vi "ProyectoBioCuinique Alpha 4.0.vi"() -> ()   [LabVIEW 2021]
uses:
  <vilib>/Utility/NIReport.llb/Report Type.ctl
  <extravilib>/ChannelInstances/Tag-dbl/Read With Abort.vi
  <extravilib>/ChannelInstances/Tag-bool/Read With Abort.vi
  <extravilib>/ChannelInstances/Tag-bool/Write With Abort.vi
  <extravilib>/ChannelInstances/Tag-dbl/Write With Abort.vi
  <vilib>/Instr/_visa.llb/VISA Configure Serial Port (Instr).vi
  <vilib>/MakerHub/LINX/Public/Utilities/Open Serial.vi
  <extravilib>/ChannelInstances/Tag-dbl/Instantiate.vi
  <extravilib>/ChannelInstances/Tag-bool/Instantiate.vi
  <extravilib>/ChannelInstances/Tag-dbl/EndpointRead.vi
  <vilib>/addons/_office/excel.llb/Excel Easy Table (str).vi
  <extravilib>/ChannelInstances/Tag-bool/EndpointRead.vi
  <extravilib>/ChannelInstances/Tag-bool/Endpoint.vi
  <extravilib>/ChannelInstances/Tag-dbl/Endpoint.vi
  <vilib>/Utility/NIReport.llb/NI_report.lvclass
  <vilib>/LabVIEW Interface for Arduino/LabVIEW Interface for Arduino.lvlib
  <vilib>/MakerHub/LINX/LMH-LINX.lvlib
  <vilib>/Utility/NIReport.llb/NI_ReportGenerationCore.lvlib
  <vilib>/addons/_office/NI_ReportGenerationToolkit.lvlib
  <vilib>/Utility/NIReport.llb/Excel/NI_Excel.lvclass
  <vilib>/MakerHub/LINX/Public/Sensors/Distance/Ultrasonic/Ultrasonic.lvlib
  <extravilib>/ChannelInstances/Tag-bool.lvlib
  <extravilib>/ChannelInstances/Tag-dbl.lvlib
panel:
  out "HUMEDAD SUELO":dbl(knob) scale=0.0..255.0
  out "TEMPERATURA":dbl(slide) scale=0.0..100.0
  out "HUMEDAD SUELO":dbl
  in  "Serial Port":refnum<visa-resource-name>="N/A"
  in  "template (empty)":path
  in  "Pin Bomba 1":u8
  in  "Pin Valvula 1":u8
  in  "Pin Valvula 2":u8
  out "HUMEDAD RELATIVA":dbl
  in  "VISA resource name":refnum<visa-resource-name>
  out "TEMPERATURA":dbl
  out "HUMEDAD RELATIVA":dbl(knob) scale=0.0..255.0
  out "Centimeters":dbl
  out "Slide":dbl(slide) scale=0.0..500.0
  out "BOMBA (11)":bool
  in  "Boolean 4":bool
  out "VALVULA (6)":bool
  in  "Boolean":bool
  out "VALVULA (5)":bool
  in  "stop":bool
  in  "VISA resource":refnum<visa-resource-name>
  # "VÁLVULA 1"
  # "BOMBA DE AGUA"
  # "VÁLVULA 2"
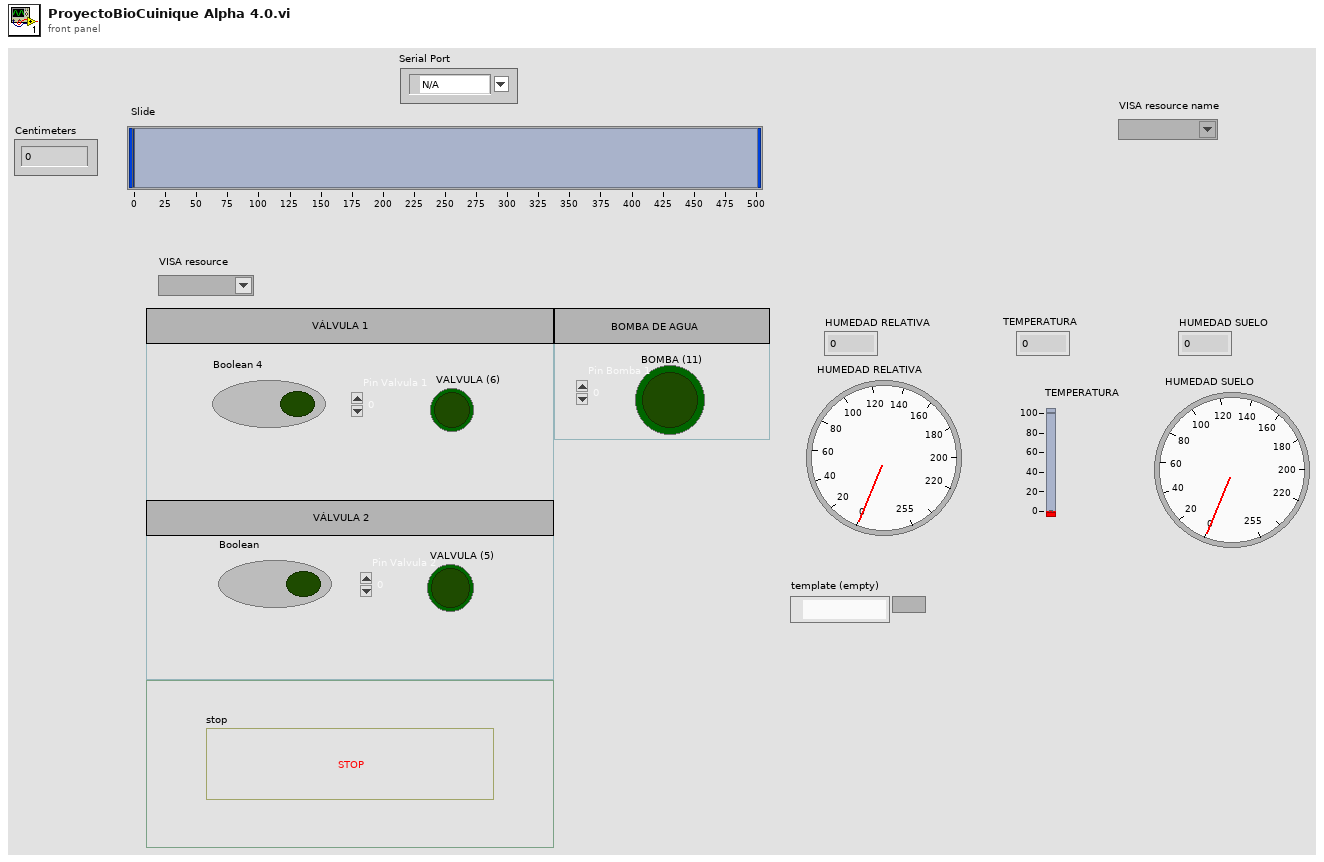
[diagram p1: front panel]
types:
  T1 = typedef "NI_ReportGenerationCore.lvlib/Report Type.ctl" = enum16{"HTML", "Word", "Excel"}
  T2 = typedef "LabVIEW Interface for Arduino.lvlib/Arduino Resource.ctl" = cluster{"VISA resource":refnum<visa-resource-name>, "Board Type":T3, "Connection Type":enum8{"USB / Serial"}, "Bytes Per Packet (15)":u8}
  T3 = typedef "LabVIEW Interface for Arduino.lvlib/Board Type.ctl" = enum16{"Uno", "Dimuelanove w/Atmega 328", "Mega 2560"}
  T4 = typedef "LMH-LINX.lvlib/LINX Ref.ctl" = cluster{"IO":T5, "Interface":T6, "LINX Device Config":T7}
  T5 = typedef "LMH-LINX.lvlib/Platform.ctl" = enum16{"Remote", "Local"}
  T6 = typedef "LMH-LINX.lvlib/Interface.ctl" = enum16{"Serial", "TCP"}
  T7 = typedef "LMH-LINX.lvlib/Device.lvlib/LINX Device Config.ctl" = cluster{"Interface":T6, "COM Port":refnum<visa-resource-name>, "TCP Configuration":T8, "Device Family":u8, "Device ID":u8, "Device Name":string, "TCP Ref":refnum<k5>, "Channels":T9}
  T8 = typedef "LMH-LINX.lvlib/Device.lvlib/TCP Config.ctl" = cluster{"IP Address":string, "Port":u16}
  T9 = typedef "LMH-LINX.lvlib/Channels.ctl" = cluster{"DI":u8[], "DO":u8[], "AI":u8[], "AO":u8[], "PWM":u8[], "QE":u8[], "UART":u8[], "I2C 2":u8[], "SPI":u8[], "CAN":u8[], "Servo":u8[], "AI Ref (V)":dbl, "AI Resolution (Bits)":u8, "AO Ref (V)":dbl, "AO Resolution (Bits)":u8}
  T10 = typedef "Tag-dbl.lvlib/))Channel.ctl" = refnum<queue>
  T11 = typedef "Tag-bool.lvlib/))Channel.ctl" = refnum<queue>
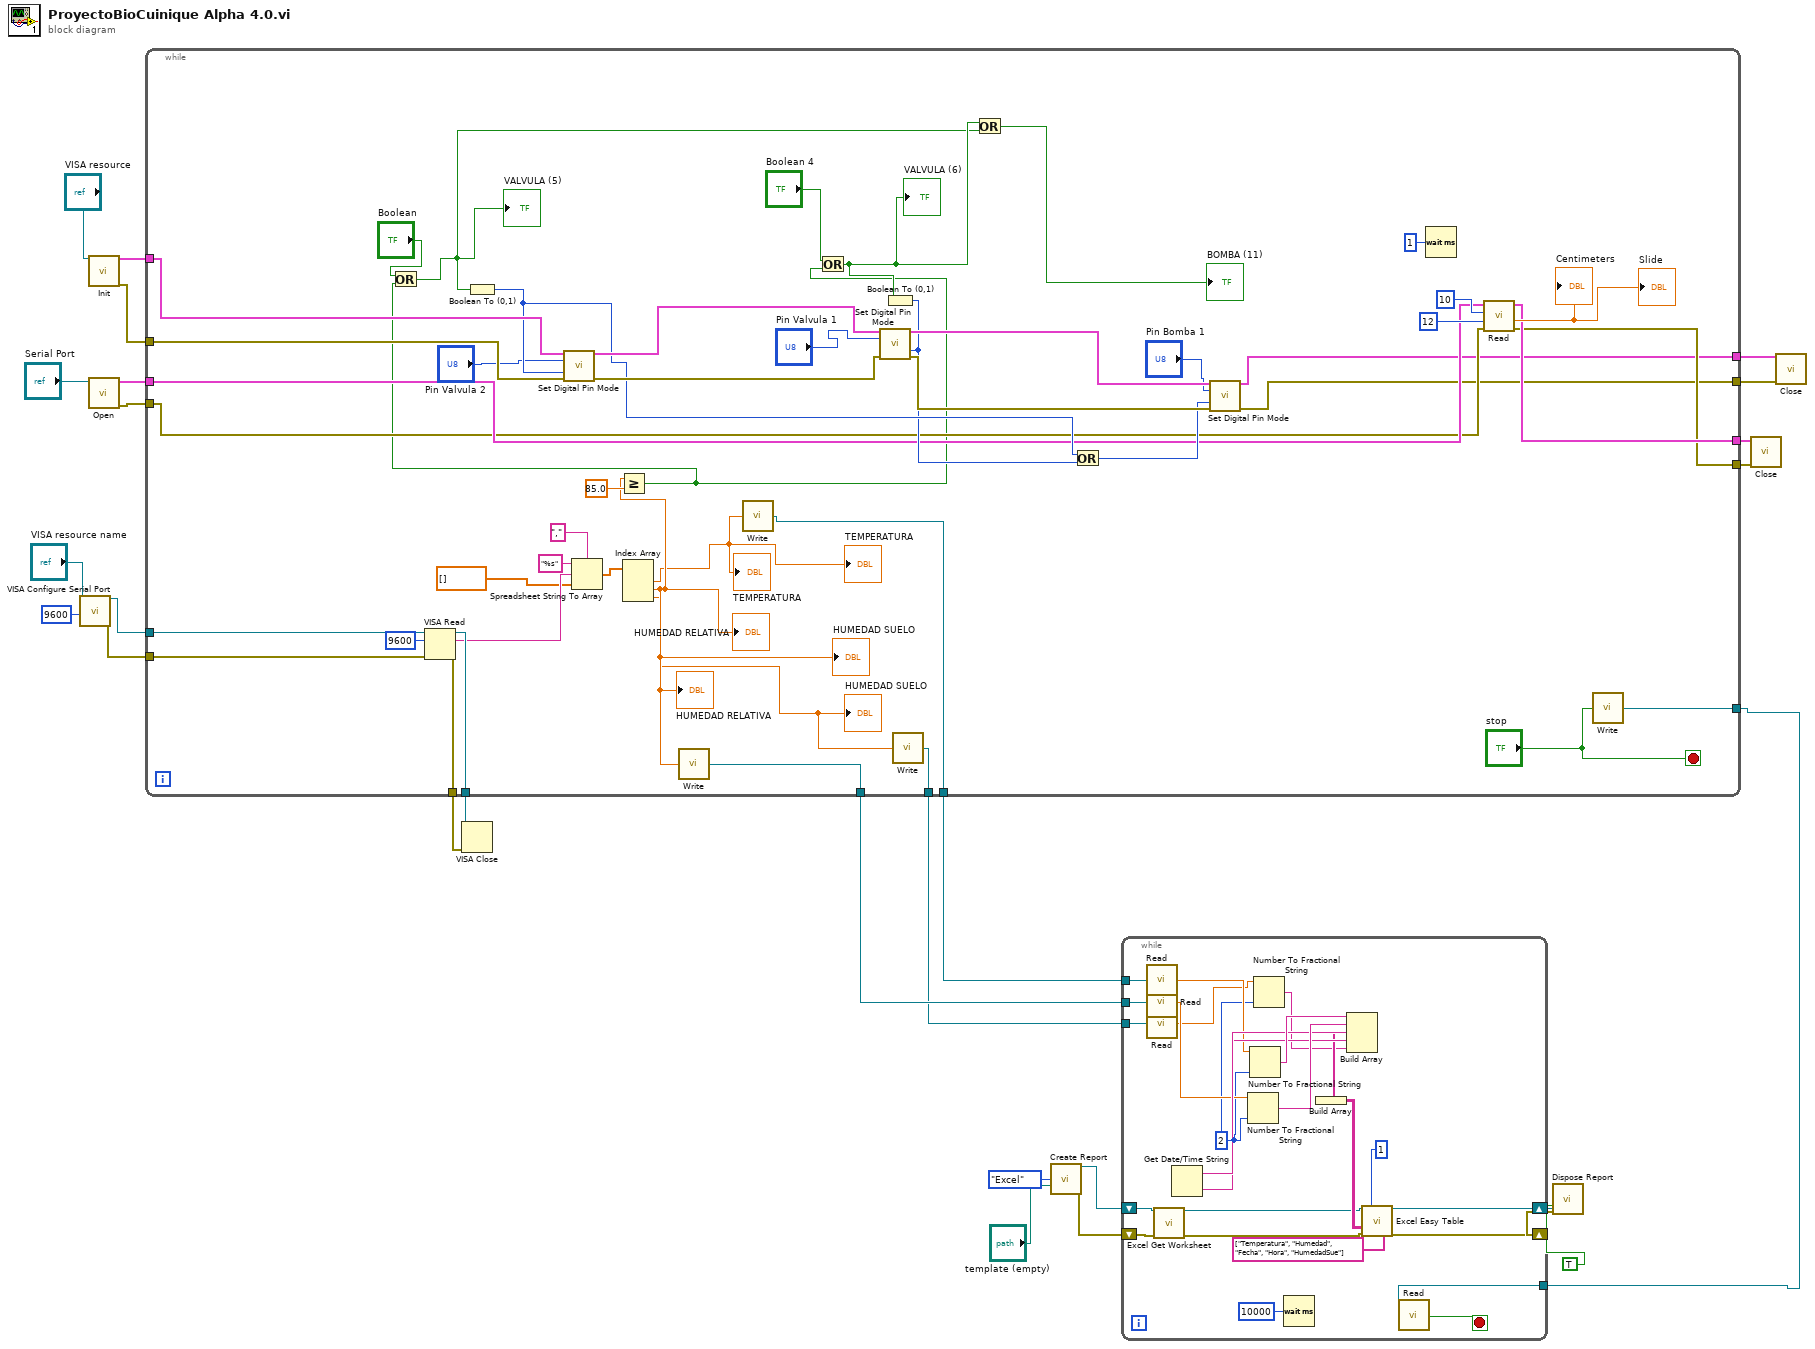
[diagram p0: block diagram]
diagram:
  n1 = call-poly "VISA Configure Serial Port"("VISA resource name"="VISA resource name", "baud rate (9600)"=u32 9600) -> ("VISA resource name out"=w18:refnum<visa-resource-name>, "error out"=w15:errorcluster)  [unwired: 12 in]
  n2 = call <vilib>:"Init.vi"("VISA resource"="VISA resource") -> ("Arduino Resource"=w26:T2, "error out"=w25:errorcluster)  [unwired: 17 in]
  n3 = call-poly <vilib>:"Open.vi"("Serial Port"="Serial Port") -> ("Error Out"=w24:errorcluster, "LINX Resource"=w23:T4)  [unwired: 8 in, 1 out]
  n4 = while {
    tunnel: w26 -> [w74]
    tunnel: w25 -> [w73]
    tunnel: w24 -> [w59]
    tunnel: w23 -> [w60]
    tunnel: [w58] -> w22
    tunnel: [w57] -> w21
    tunnel: [w56] -> w20
    tunnel: [w55] -> w19
    tunnel: w18 -> [w54]
    tunnel: [w53] -> w17
    tunnel: [w52] -> w16
    tunnel: w15 -> [w51]
    tunnel: [w36] -> w5
    tunnel: [w35] -> w4
    tunnel: [w34] -> w3
    tunnel: [w28] -> w1
    stop <- "stop" stop-if-true
    n5 = VISA Read(VISA resource name=w54, byte count=u32 9600, error in (no error)=w51) -> (VISA resource name out=w52:refnum<visa-resource-name>, read buffer=w50:string, error out=w53:errorcluster)  [unwired: 1 out]
    n6 = Spreadsheet String To Array(delimiter (Tab)=",", format string="%s", spreadsheet string=w50, array type (2D Dbl)=dbl[] []) -> (array=w46:dbl[])
    n7 = Index Array(array=w46) -> (element #1=w30:dbl, element #2=w43:dbl, element #3=w29:dbl)  [unwired: 3 in]
    "HUMEDAD RELATIVA" <- w43
    "TEMPERATURA" <- w30
    "HUMEDAD RELATIVA" <- w43
    "HUMEDAD SUELO" <- w29
    "TEMPERATURA" <- w30
    "HUMEDAD SUELO" <- w29
    n8 = Greater Or Equal?(x=w43, y=85.0) -> (x >= y?=w33:bool)
    n9 = Or(x="Boolean", y=w33) -> (x .or. y?=w31:bool)
    "VALVULA (5)" <- w31
    n10 = Boolean To (0,1)(Boolean=w31) -> (0, 1=w68:i16)
    n11 = call <vilib>:"Set Digital Pin Mode.vi"("Arduino Resource"=w74, "Digital I/O Pin"="Pin Valvula 2", "Pin Mode (Input)"=w68, "error in"=w73) -> ("Arduino Resource"=w72:T2, "error out"=w71:errorcluster)  [unwired: 10 in]
    n12 = call <extravilib>:"Write.vi"("element"=w43) -> ("channel"=w34:T10)  [unwired: 1 out]
    n13 = call <extravilib>:"Write.vi"("element"=w30) -> ("channel"=w35:T10)  [unwired: 1 out]
    n14 = Or(x="Boolean 4", y=w33) -> (x .or. y?=w41:bool)
    "VALVULA (6)" <- w41
    n15 = Boolean To (0,1)(Boolean=w41) -> (0, 1=w67:i16)
    n16 = call <vilib>:"Set Digital Pin Mode.vi"("Arduino Resource"=w72, "Digital I/O Pin"="Pin Valvula 1", "Pin Mode (Input)"=w67, "error in"=w71) -> ("Arduino Resource"=w69:T2, "error out"=w70:errorcluster)  [unwired: 10 in]
    n17 = call <extravilib>:"Write.vi"("element"=w29) -> ("channel"=w28:T10)  [unwired: 1 out]
    n18 = Or(x=w41, y=w31) -> (x .or. y?=→"BOMBA (11)":bool)
    n19 = Or(x=w68, y=w67) -> (x .or. y?=w66:i16)
    n20 = call <vilib>:"Set Digital Pin Mode.vi"("Arduino Resource"=w69, "Digital I/O Pin"="Pin Bomba 1", "Pin Mode (Input)"=w66, "error in"=w70) -> ("Arduino Resource"=w56:T2, "error out"=w55:errorcluster)  [unwired: 10 in]
    n21 = Wait (ms)(milliseconds to wait=u32 1) -> ()  [unwired: 1 out]
    n22 = call <vilib>:"Read.vi"("Error In"=w59, "DO Channel"=u8 12, "DI Channel"=u8 10, "LINX Resource"=w60) -> ("Error Out"=w57:errorcluster, "Centimeters"=→"Centimeters" →"Slide":dbl, "LINX Resource"=w58:T4)  [unwired: 4 in, 1 out]
    n23 = call <extravilib>:"Write.vi"("element"="stop") -> ("channel"=w36:T11)  [unwired: 1 out]
  }
  n24 = VISA Close(VISA resource name=w16, error in (no error)=w17) -> ()  [unwired: 1 out]
  n25 = call <vilib>:"Create Report.vi"("report type"=Report_Type."Excel", "template (empty)"="template (empty)") -> ("report out"=w9:refnum<class "NI_report.lvclass">, "error out"=w10:errorcluster)  [unwired: 12 in]
  n26 = while {
    shift-right: [w88] -> w7
    shift-left: w10 -> [w93]
    shift-right: [w89] -> w8
    shift-left: w9 -> [w91]
    tunnel: w5 -> [w84]
    tunnel: w4 -> [w82]
    tunnel: w3 -> [w80]
    tunnel: w1 -> [w78]
    stop <- w83 stop-if-true
    w77 = i16 2 ("precision (6)")
    n27 = call <vilib>:"Read.vi"("channel"=w82) -> ("element"=w81:dbl)  [unwired: 1 in, 1 out]
    n28 = call <vilib>:"Read.vi"("channel"=w80) -> ("element"=w79:dbl)  [unwired: 1 in, 1 out]
    n29 = call <vilib>:"Read.vi"("channel"=w78) -> ("element"=w76:dbl)  [unwired: 1 in, 1 out]
    n30 = call <vilib>:"Excel Get Worksheet.vi"("report in"=w91, "error in (no error)"=w93) -> ("report out"=w90:refnum<class "NI_report.lvclass">, "error out"=w92:errorcluster)  [unwired: 12 in]
    n31 = Get Date/Time String() -> (date string=w97:string, time string=w96:string)  [unwired: 3 in]
    n32 = Number To Fractional String(number=w79, precision (6)=w77) -> (F-format string=w98:string)  [unwired: 2 in]
    n33 = Number To Fractional String(number=w81, precision (6)=w77) -> (F-format string=w99:string)  [unwired: 2 in]
    n34 = Number To Fractional String(number=w76, precision (6)=w77) -> (F-format string=w75:string)  [unwired: 2 in]
    n35 = Wait (ms)(milliseconds to wait=u32 10000) -> ()  [unwired: 1 out]
    n36 = Build Array(w99, w98, w97, w96, w75) -> (w95:string[])
    n37 = Build Array(w95) -> (w94:string[][])
    n38 = call-poly <vilib>:"Excel Easy Table.vi"("report in"=w90, "iteration"=1, "text data"=w94, "error in (no error)"=w92, "column headers"=string[] ["Temperatura", "Humedad", "Fecha", "Hora", "HumedadSue"]) -> ("report out"=w89:refnum<class "NI_report.lvclass">, "error out"=w88:errorcluster)  [unwired: 6 in, 3 out]
    n39 = call <vilib>:"Read.vi"("channel"=w84) -> ("element"=w83:bool)  [unwired: 1 in, 1 out]
  }
  n40 = call-dynamic "Dispose Report.vi"("report in"=w8, "save changes? (F)"=TRUE, "error in (no error)"=w7) -> ()  [unwired: 12 in, 1 out]
  n41 = call <vilib>:"Close.vi"("Error In"=w21, "LINX Resource"=w22) -> ()  [unwired: 9 in, 1 out]
  n42 = call <vilib>:"Close.vi"("Arduino Resource"=w20, "error in"=w19) -> ()  [unwired: 13 in, 1 out]
